vi "Excel Cell Address to Numeric Indices.vi"(11 "Cell Name":string) -> (2 "Row Number":i32, 3 "Column Number":i32)   [LabVIEW 2019, in "Open Xml.lvlib"]
doc: "Converts an Excel Column Letter String to the numeric column count. This handles AB greater than 25 column callouts. Excel column count is 0 based.\nJack Hamilton\nC6 Systems, Inc C6Systems.com\nFree to use and distribute"
uses:
  Open Xml.lvlib
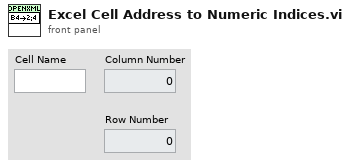
[diagram p1: front panel]
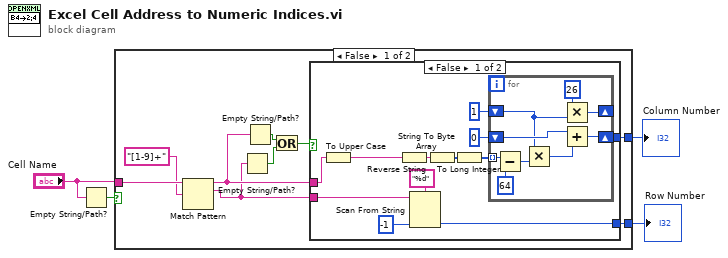
[diagram p0: block diagram]
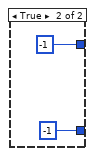
[diagram p2: hidden frame]
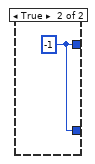
[diagram p3: hidden frame]
diagram:
  n1 = Empty String/Path?(string/path="Cell Name") -> (empty?=w2:bool)
  n2 = case shown="False" w2 {
    tunnel: [w13 w37] -> w4
    tunnel: "Cell Name" -> [w12 _]
    tunnel: [w11 w37] -> w3
    frame False {
      n3 = Match Pattern(string=w12, regular expression="[1-9]+") -> (before substring=w7:string, match substring=w5:string)  [unwired: 1 in, 2 out]
      n4 = Empty String/Path?(string/path=w5) -> (empty?=w6:bool)
      n5 = Empty String/Path?(string/path=w7) -> (empty?=w8:bool)
      n6 = Or(x=w8, y=w6) -> (x .or. y?=w9:bool)
      n7 = case shown="False" w9 {
        tunnel: [w20 -1] -> w13
        tunnel: [w16 -1] -> w11
        tunnel: w7 -> [w15 _]
        tunnel: w5 -> [w14 _]
        frame False {
          n8 = To Upper Case(1:w15) -> (0:w21:string)
          n9 = Reverse String(1:w21) -> (0:w23:string)
          n10 = Scan From String(format string="%d" ("Format String"), input string=w14, default 1=-1) -> (output 1=w16:i32)  [unwired: 2 in, 3 out]
          n11 = String To Byte Array(string=w23) -> (unsigned byte array=w22:u8[])
          n12 = To Long Integer(number=w22) -> (32bit integer=w17:i32[])
          n13 = for {
            tunnel: w17 -> [w34] mode=indexing
            shift-right: [w30] -> w20
            shift-left: 0 -> [w27]
            shift-right: [w32] -> _
            shift-left: 1 -> [w26]
            n14 = Subtract(x=w34, y=64) -> (x-y=w28:i32)
            n15 = Multiply(x=w26, y=w28) -> (x*y=w29:i32)
            n16 = Multiply(x=26, y=w26) -> (x*y=w32:i32)
            n17 = Add(x=w27, y=w29) -> (x+y=w30:i32)
          }
        }
        frame True {
        }
      }
    }
    frame True {
      w37 = -1
    }
  }
  "Row Number" <- w3
  "Column Number" <- w4
